vi "Calculate Index Interleaved Array.vi"(6 "Index":i32, 8 "Buffer Wrap Around":bool, 9 "Number of Channels":u32, 10 "Interleaved Array":sgl[](array[numeric]), 11 "Position Zero":u32) -> (3 "Array":sgl[](array[numeric]))   [LabVIEW 2014]
uses:
  <userlib>/_OpenG.lib/array/array.llb/Index 1D Array Elements (SGL)__ogtk.vi
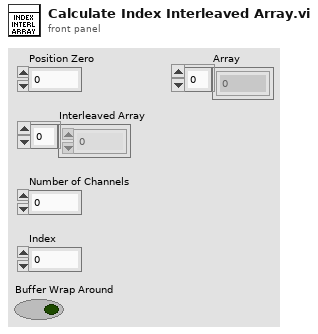
[diagram p1: front panel]
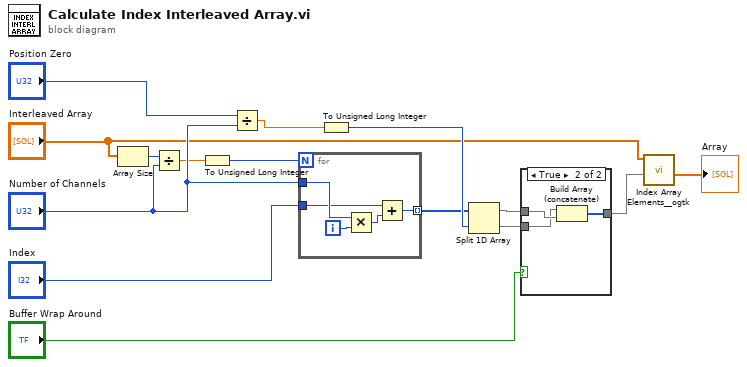
[diagram p0: block diagram]
diagram:
  n1 = Array Size(array="Interleaved Array") -> (size(s)=w4:i32)
  n2 = Divide(x=w4, y="Number of Channels") -> (x/y=w5:dbl)
  n3 = To Unsigned Long Integer(number=w5) -> (unsigned 32bit integer=w6:u32)
  n4 = Divide(x="Position Zero", y="Number of Channels") -> (x/y=w10:dbl)
  n5 = for {
    N: w6 -> [_]
    tunnel: "Index" -> [w17]
    tunnel: "Number of Channels" -> [w19]
    tunnel: [w16] -> w7 mode=indexing
    i -> [w20]
    n6 = Multiply(x=w19, y=w20) -> (x*y=w18:u32)
    n7 = Add(x=w17, y=w18) -> (x+y=w16:u32)
  }
  n8 = To Unsigned Long Integer(number=w10) -> (unsigned 32bit integer=w11:u32)
  n9 = Split 1D Array(array=w7, index=w11) -> (first subarray=w13:u32[], second subarray=w12:u32[])
  n10 = case shown="True" "Buffer Wrap Around" {
    tunnel: [w21 w24] -> w14
    tunnel: w13 -> [w21 w23]
    tunnel: w12 -> [_ w22]
    frame False {
    }
    frame True {
      n11 = Build Array (concatenate)(w22, w23) -> (w24:u32[])
    }
  }
  n12 = call-poly <userlib>:"Index Array Elements__ogtk.vi"("indices"=w14, "array"="Interleaved Array") -> ("elements"=→"Array":sgl[])  [unwired: 9 in]
